vi "SyncMissions.vi"(11 "Mission Notifiers":T1) -> (3 "Mission Notifiers OUT":T1)   [LabVIEW 2013]
doc: "This VI checks whether there are any new Finished Missions. If so, it checks them off in the Mission Array.\n\nEric Schneider, August 2014"
uses:
  Data/TypeDefs/MissionNotifiers.ctl
  Classes/Missions/GenericMission/GenericMission.lvclass
  Classes/Obstacle/Obstacle.lvclass
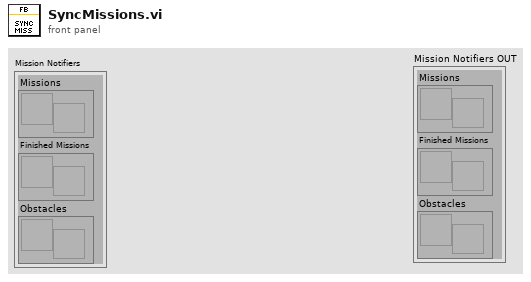
[diagram p1: front panel]
types:
  T1 = typedef "MissionNotifiers.ctl" = cluster{"Missions":refnum<notifier>, "Finished Missions":refnum<notifier>, "Obstacles":refnum<notifier>}
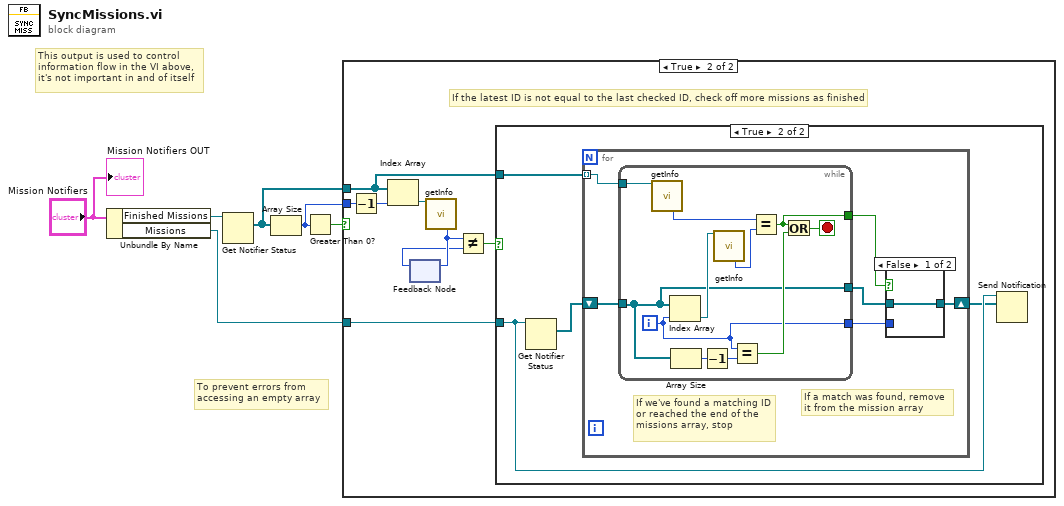
[diagram p0: block diagram]
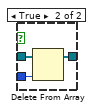
[diagram p4: hidden frame]
diagram:
  # "To prevent errors from accessing an empty array"
  # "This output is used to control information flow in the VI above, it's not important in and of itself"
  n1 = Unbundle By Name("Mission Notifiers") -> ("Finished Missions"=w6:refnum<notifier>, "Missions"=w1:refnum<notifier>)
  n2 = Get Notifier Status(notifier=w6) -> (current notification=w2:refnum<class "GenericMission.lvclass">[])  [unwired: 1 in, 4 out]
  n3 = Array Size(array=w2) -> (size(s)=w3:i32)
  n4 = Greater Than 0?(x=w3) -> (x > 0?=w4:bool)
  n5 = case shown="True" w4 {
    tunnel: w3 -> [_ w14]
    tunnel: w2 -> [_ w7]
    tunnel: w1 -> [_ w8]
    frame False {
    }
    frame True {
      # "If the latest ID is not equal to the last checked ID, check off more missions as finished"
      n6 = Decrement(x=w14) -> (x-1=w13:i32)
      n7 = Index Array(array=w7, index=w13) -> (element=w12:refnum<class "GenericMission.lvclass">)
      n8 = feedback #1() -> (w10:i16)  [unwired: 1 in]
      n9 = call-dynamic "getInfo.vi"("GenericMission in"=w12) -> ("ID#"=w11:i16)  [unwired: 6 in, 8 out]
      n10 = feedback-in #1(w11) -> ()
      n11 = Not Equal?(x=w11, y=w10) -> (x != y?=w9:bool)
      n12 = case shown="True" w9 {
        tunnel: w8 -> [_ w16]
        tunnel: w7 -> [_ w18]
        frame False {
        }
        frame True {
          n13 = Get Notifier Status(notifier=w16) -> (current notification=w17:refnum<class "GenericMission.lvclass">[])  [unwired: 1 in, 4 out]
          n14 = for {
            tunnel: w18 -> [w23] mode=indexing
            shift-right: [w20] -> w15
            shift-left: w17 -> [w24]
            # "If we've found a matching ID or reached the end of the missions array, stop"
            # "If a match was found, remove it from the mission array"
            n15 = while {
              tunnel: w24 -> [w31]
              tunnel: w23 -> [w39]
              tunnel: [w31] -> w22
              tunnel: [w30] -> w21
              tunnel: [w29] -> w19
              i -> [w30]
              stop <- w35 stop-if-true
              n16 = call-dynamic "getInfo.vi"("GenericMission in"=w39) -> ("ID#"=w36:i16)  [unwired: 6 in, 8 out]
              n17 = Index Array(array=w31, index=w30) -> (element=w38:refnum<class "GenericMission.lvclass">)
              n18 = Array Size(array=w31) -> (size(s)=w34:i32)
              n19 = Decrement(x=w34) -> (x-1=w33:i32)
              n20 = call-dynamic "getInfo.vi"("GenericMission in"=w38) -> ("ID#"=w37:i16)  [unwired: 6 in, 8 out]
              n21 = Equal?(x=w30, y=w33) -> (x = y?=w32:bool)
              n22 = Equal?(x=w36, y=w37) -> (x = y?=w29:bool)
              n23 = Or(x=w29, y=w32) -> (x .or. y?=w35:bool)
            }
            n24 = case shown="False" w19 {
              tunnel: w22 -> [w25 w28]
              tunnel: w21 -> [_ w27]
              tunnel: [w25 w26] -> w20
              frame False {
              }
              frame True {
                n25 = Delete From Array(array=w28, index=w27) -> (array with subset deleted=w26:refnum<class "GenericMission.lvclass">[])  [unwired: 1 in, 1 out]
              }
            }
          }
          n26 = Send Notification(notification=w15, notifier=w16) -> ()  [unwired: 1 in, 2 out]
        }
      }
    }
  }
  "Mission Notifiers OUT" <- "Mission Notifiers"
